vi "Global Setup.vi"(8 "error in (no error)":errorcluster, 11 "Demo Test in":refnum<class "Global Fixture Demo Test Case.lvclass">) -> (0 "error out":errorcluster)   [LabVIEW 2020, in "Global Fixture Demo Test Case.lvclass"]
uses:
  Global Fixture Demo Test Case.lvclass
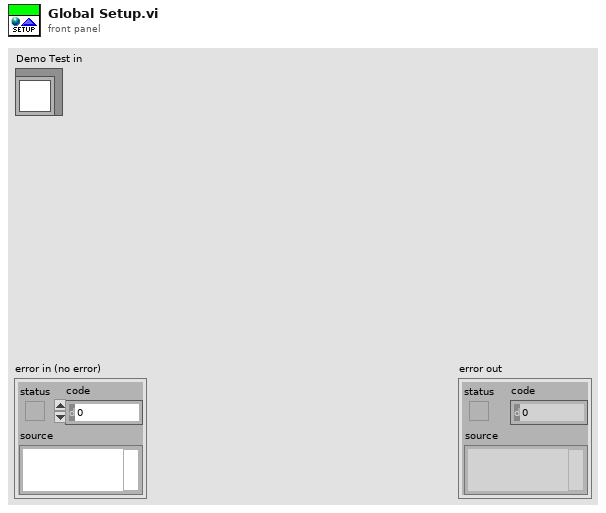
[diagram p1: front panel]
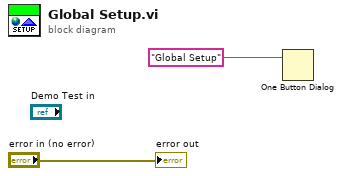
[diagram p0: block diagram]
diagram:
  n1 = One Button Dialog(message="Global Setup") -> ()  [unwired: 1 in, 1 out]
  "error out" <- "error in (no error)"
